vi "Configure Event Search (Serial Bus - CAN).vi"(5 "ID Value Type (0: Standard)":i32(ring) items=["Standard", "Extended"], 6 "ID Value (0xXXX)":string="0xXXX", 7 "Data Length (4)":dbl=4.0, 8 "error in (no error)":errorcluster, 9 "Data (0xXX)":string="0xXX", 10 "Search Operation (0: Data)":i32(ring) items=["Data", "ID Data", "ID Either", "ID Remote", "All Errors", "Overload", "Error"], 11 "VISA resource name":refnum<visa-resource-name>) -> (0 "error out":errorcluster, 3 "VISA resource name out":refnum<visa-resource-name>)   [LabVIEW 2015, in "Agilent 2000 3000 X-Series.lvlib"]
doc: "Configures the event search of CAN bus."
uses:
  <instrlib>/Agilent 2000 3000 X-Series/Agilent 2000 3000 X-Series.lvlib
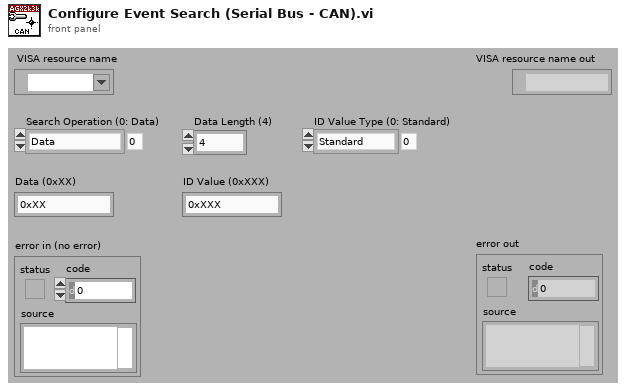
[diagram p1: front panel]
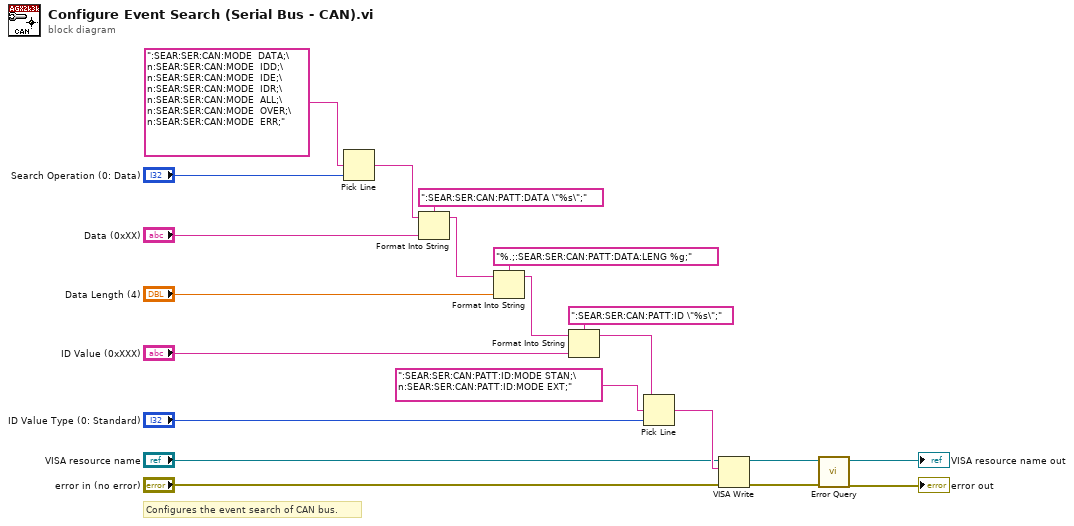
[diagram p0: block diagram]
diagram:
  # "Configures the event search of CAN bus."
  n1 = Pick Line(multi-line string=":SEAR:SER:CAN:MODE  DATA;\n:SEAR:SER:CAN:MODE  IDD;\n:SEAR:SER:CAN:MODE  IDE;\n:SEAR:SER:CAN:MODE  IDR;\n:SEAR:SER:CAN:MODE  ALL;\n:SEAR:SER:CAN:MODE  OVER;\n:SEAR:SER:CAN:MODE  ERR;", line index="Search Operation (0: Data)") -> (output string=w19:string)  [unwired: 1 out]
  n2 = Format Into String(format string=":SEAR:SER:CAN:PATT:DATA \"%s\";", initial string=w19, "Data (0xXX)") -> (resulting string=w16:string)  [unwired: 1 in, 1 out]
  n3 = Format Into String(format string="%.;:SEAR:SER:CAN:PATT:DATA:LENG %g;", initial string=w16, "Data Length (4)") -> (resulting string=w13:string)  [unwired: 1 in, 1 out]
  n4 = Format Into String(format string=":SEAR:SER:CAN:PATT:ID \"%s\";", initial string=w13, "ID Value (0xXXX)") -> (resulting string=w8:string)  [unwired: 1 in, 1 out]
  n5 = Pick Line(string ("")=w8, multi-line string=":SEAR:SER:CAN:PATT:ID:MODE STAN;\n:SEAR:SER:CAN:PATT:ID:MODE EXT;", line index="ID Value Type (0: Standard)") -> (output string=w7:string)
  n6 = VISA Write(VISA resource name="VISA resource name", write buffer=w7, error in (no error)="error in (no error)") -> (VISA resource name out=w4:refnum<visa-resource-name>, error out=w3:errorcluster)  [unwired: 1 out]
  n7 = call <instrlib>:"Error Query.vi"("error in (no error)"=w3, "VISA resource name"=w4) -> ("error out"=→"error out":errorcluster, "VISA resource name out"=→"VISA resource name out":refnum<visa-resource-name>)  [unwired: 8 out]
